vi "start-stop-exit.vi"(8 "Exit":bool, 9 "stop":bool, 10 "start":bool, 11 "current-state":T1) -> (3 "new-state":T1)   [LabVIEW 2024]
uses:
  state-enum.ctl
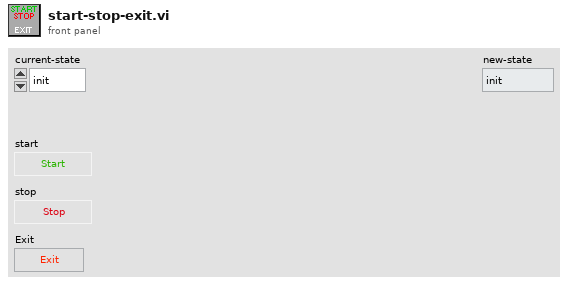
[diagram p1: front panel]
types:
  T1 = typedef "state-enum.ctl" = enum16{"init", "wait", "start", "run", "stop", "exit"}
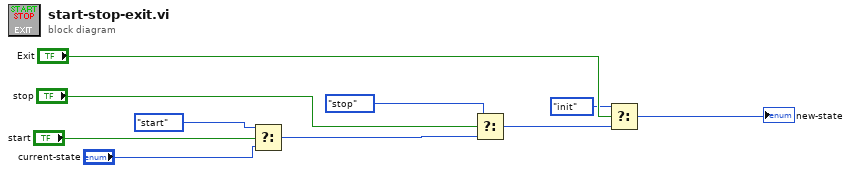
[diagram p0: block diagram]
diagram:
  n1 = Select(t=state-enum."start", s="start", f="current-state") -> (s? t:f=w8:T1)
  n2 = Select(t=state-enum."stop", s="stop", f=w8) -> (s? t:f=w4:T1)
  n3 = Select(t=state-enum."init", s="Exit", f=w4) -> (s? t:f=→"new-state":T1)
